vi "Actor Core.vi"(8 "error in (no error)":errorcluster, 11 "Mag Lab Measure Interface in":refnum<class "Thermopower UI.lvclass">) -> (0 "error out":errorcluster, 3 "Actor Framework.lvlib:Actor":refnum<class "Actor.lvclass">)   [LabVIEW 2015, in "Thermopower UI.lvclass"]
uses:
  Thermopower UI.lvclass
  <vilib>/ActorFramework/Actor/Actor.lvclass
  Queued Listbox/Queued Listbox.xctl
  Controls/Menu object.ctl
  <vilib>/ActorFramework/Actor/Actor.lvclass/Actor.ctl
  <vilib>/ActorFramework/Message Enqueuer/Message Enqueuer.lvclass/Message Enqueuer.ctl
  Mag Lab Measure Base Messages/Open sub-object parameters Msg/Open nested object parameters Msg.lvclass/Open nested object parameters Msg.ctl
  <vilib>/ActorFramework/Message Enqueuer/Init from Existing Queue.vi
  <vilib>/ActorFramework/Message Enqueuer/Enqueue.vi
  <vilib>/ActorFramework/Message Priority Queue/Priority Enqueue.vi
  <vilib>/ActorFramework/Message Enqueuer/Message Enqueuer.lvclass
  Mag Lab Measure Base Messages/Open sub-object parameters Msg/Open nested object parameters Msg.lvclass
  <vilib>/ActorFramework/Stop Msg/Stop Msg.lvclass
  Mag Lab Measure Interface/Interface with menu/Interface with menu.lvclass
panel:
  out "Name":string
  in  "Mode of operation":enum16{""}(ring)
  in  "Heater Power Source":T1 {"Object name" items=["Select one"]}
  in  "Recorder(s)":string[](xcontrol)
  in  "Close":bool
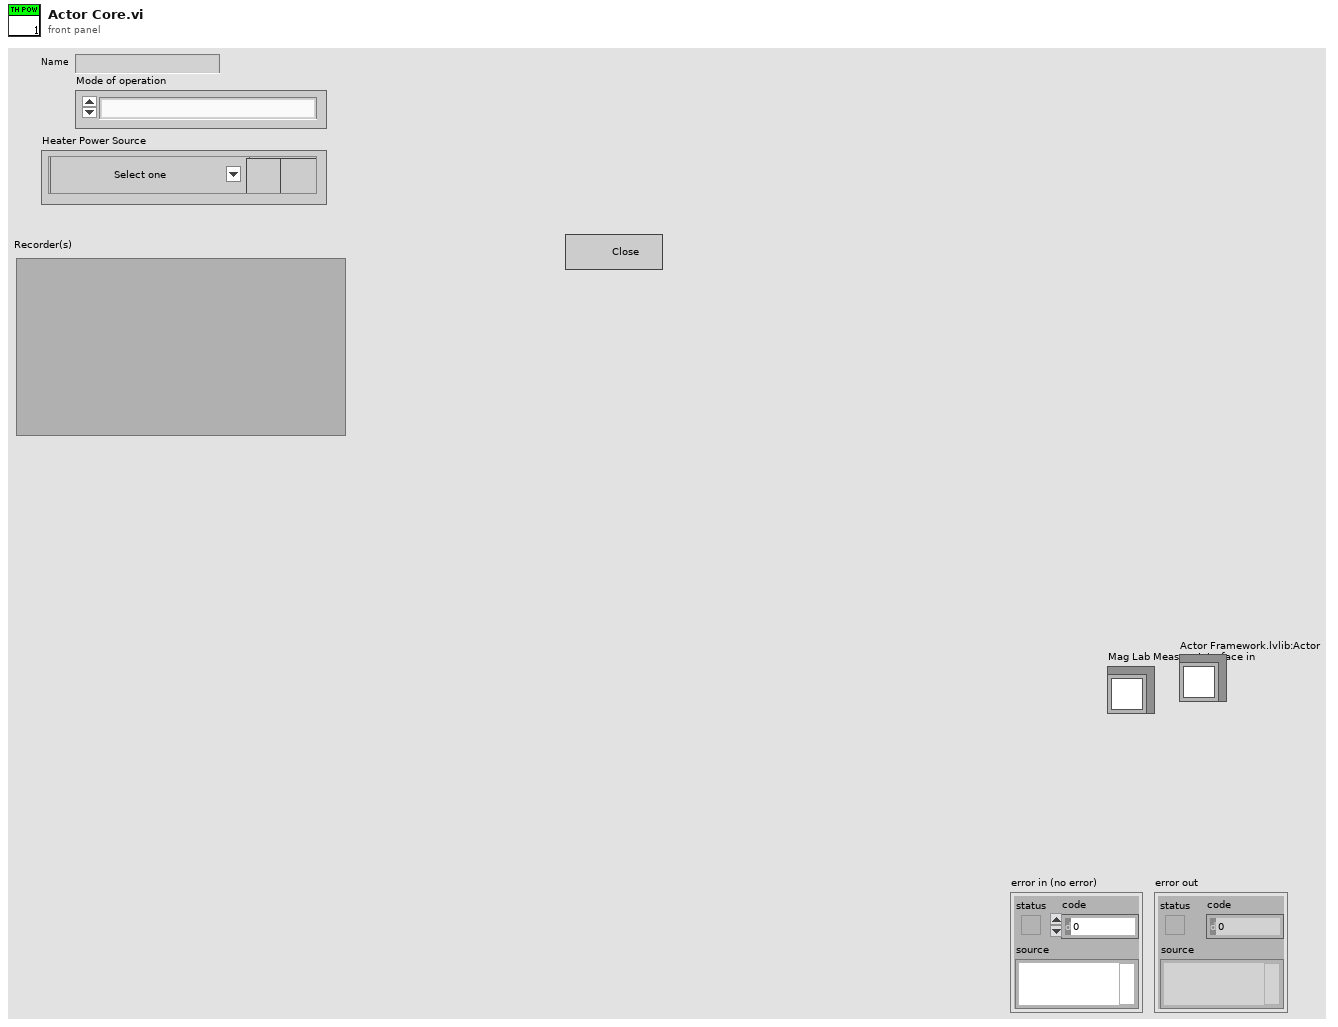
[diagram p1: front panel]
types:
  T1 = typedef "Menu object.ctl" = cluster{"Object name":u16, "Open parameters":bool, "Remove Button":bool}
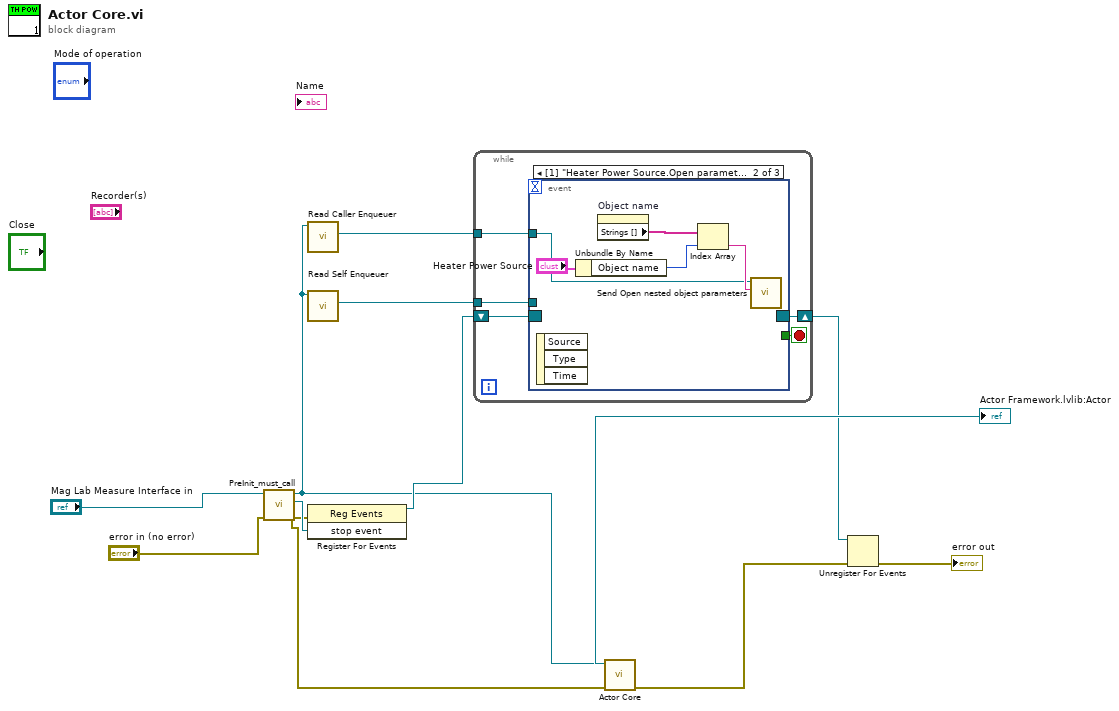
[diagram p0: block diagram]
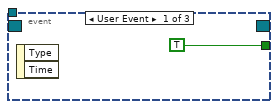
[diagram p2: hidden frame]
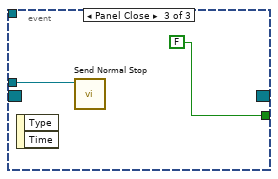
[diagram p3: hidden frame]
diagram:
  n1 = call-dynamic "PreInit_must_call.vi"("error in (no error)"="error in (no error)", "Mag Lab Measure Interface in"="Mag Lab Measure Interface in") -> ("error out"=w4:errorcluster, "stop event"=w11:refnum<user-event>, "Mag Lab Measure Interface out"=w6:refnum<class "Thermopower UI.lvclass">)  [unwired: 7 in]
  n2 = call <vilib>:"Read Caller Enqueuer.vi"("Actor"=w6) -> ("Caller Enqueuer"=w8:refnum<class "Message Enqueuer.lvclass">)  [unwired: 10 in]
  n3 = call <vilib>:"Read Self Enqueuer.vi"("Actor"=w6) -> ("Self Enqueuer"=w9:refnum<class "Message Enqueuer.lvclass">)  [unwired: 10 in]
  n4 = register-events(error in=w4, w11) -> (reference out=w10:refnum<event-registration>)  [unwired: 1 in, 1 out]
  n5 = while {
    tunnel: w9 -> [w15]
    tunnel: w8 -> [w14]
    shift-right: [w13] -> w1
    shift-left: w10 -> [w17]
    stop <- w16 stop-if-true
    n6 = event shown="[1] \"Heater Power Source.Open parameters\": Value Change" {
      selector: w17 -> [_ _ _]
      dyn-events: [_ _ _] -> w13
      timeout: _ -> [_ _ _]
      tunnel: [TRUE _ FALSE] -> w16
      tunnel: w15 -> [_ _ w24]
      tunnel: w14 -> [_ w19 _]
      event User Event {
        n7 = event-data() -> ()  [unwired: 1 in, 2 out]
      }
      event Value Change {
        n8 = event-data() -> ()  [unwired: 1 in, 3 out]
        n9 = Unbundle By Name("Heater Power Source") -> ("Object name"=w22:u16)
        n10 = property on="Object name" class="Ring (strict)"() -> ("Strings []"=w23:string[])  [unwired: 2 in, 2 out]
        n11 = Index Array(array=w23, index=w22) -> (element=w21:string)
        n12 = call "Send Open nested object parameters.vi"("Object name"=w21, "Message Enqueuer"=w19) -> ()  [unwired: 8 in, 2 out]
      }
      event Panel Close {
        n13 = event-data() -> ()  [unwired: 1 in, 2 out]
        n14 = call <vilib>:"Send Normal Stop.vi"("Message Enqueuer"=w24) -> ()  [unwired: 10 in, 1 out]
      }
    }
  }
  n15 = call-parent "Actor Core.vi"("error in (no error)"=w4, "Mag Lab Measure Interface in"=w6) -> ("error out"=w3:errorcluster, "Actor Framework.lvlib:Actor"=→"Actor Framework.lvlib:Actor":refnum<class "Actor.lvclass">)  [unwired: 8 in]
  n16 = Unregister For Events(event registration refnum=w1, error in=w3) -> (error out=→"error out":errorcluster)
